vi "MainLoop.vi"() -> ()   [LabVIEW 2021]
uses:
  5a09477c-fa6a-4a2c-ae4e-0462b0b96a3d.vi
  6f825153-6f78-4197-a3b4-cb3bcc6ce098.vi
  <vilib>/DAQmx/read.llb/DAQmx Read (Digital 1D Bool 1Chan 1Samp).vi
  <vilib>/DAQmx/create/channels.llb/DAQmx Create Channel (DI-Digital Input).vi
  <vilib>/Utility/file.llb/Read Delimited Spreadsheet (DBL).vi
  GlobalSTATE.vi
  <vilib>/DAQmx/miscellaneous.llb/DAQmx Fill In Error Info.vi
  Global_BeamBreaks.vi
  <vilib>/Utility/file.llb/Write Delimited Spreadsheet (string).vi
panel:
  in  "stop":bool
  in  "Tab Control":enum32{"Settings", "Monitor", "Events"}(tab)
  in  "Task type":T1(ring)=enum."One drive changes"
  in  "Drive to change (in 'One drive changes')":enum32{"Food", "Water", "Social"}(ring)
  in  "Possible availability":i32[](array[numeric])=[0, 1, 2]
  in  "Control availability":i32=1
  in  "Beam break digital inputs":tag="Dev2/port0/line0:4"
  in  "Availability settings":i32[][](array[numeric])=[[0, 1, 2], [0, 1, 2], [0, 4000, 8000]]
  in  "file (use dialog)":path=path "C:/Code/Availability-maze-main/Availability-maze-main/MazeCode/LookUpTbl.txt"
  in  "Beam breaks":bool[](array[boolean])=[FALSE, FALSE, FALSE, FALSE, FALSE]
  out "Current State":string="CHOICE"
  out "Block length":i32=3
  out "Max pellets":u32
  out "Interaction time (ms)":u32=4000
  out "Max water drops":u32=1
  out "Block count":i32
  out "Trial of block":i32
  out "Food available":dbl(knob) scale=0.0..3.0
  out "Water available":dbl(knob)=0.46403176085318276 scale=0.0..3.0
  out "Social time available":dbl(knob)=4000.0 scale=0.0..10000.0
  out "serial comm":string="b"
  out "Event times":string[][](array[string])
  in  "Save event file?":bool
  in  "file path (dialog if empty)":path
  # "Low (0)     Medium (1)    High(2)"
  # "Pellets \n\nWater drops\n\nSocial time (ms)"
  # "Social                   Water                  Food               Middle             Home cage"
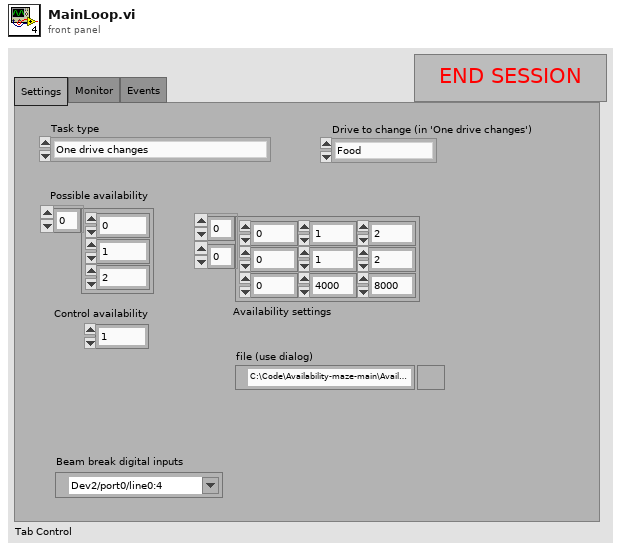
[diagram p1: front panel]
types:
  T1 = enum32{"All drives change and different", "One drive changes", "All drives same, but change"}
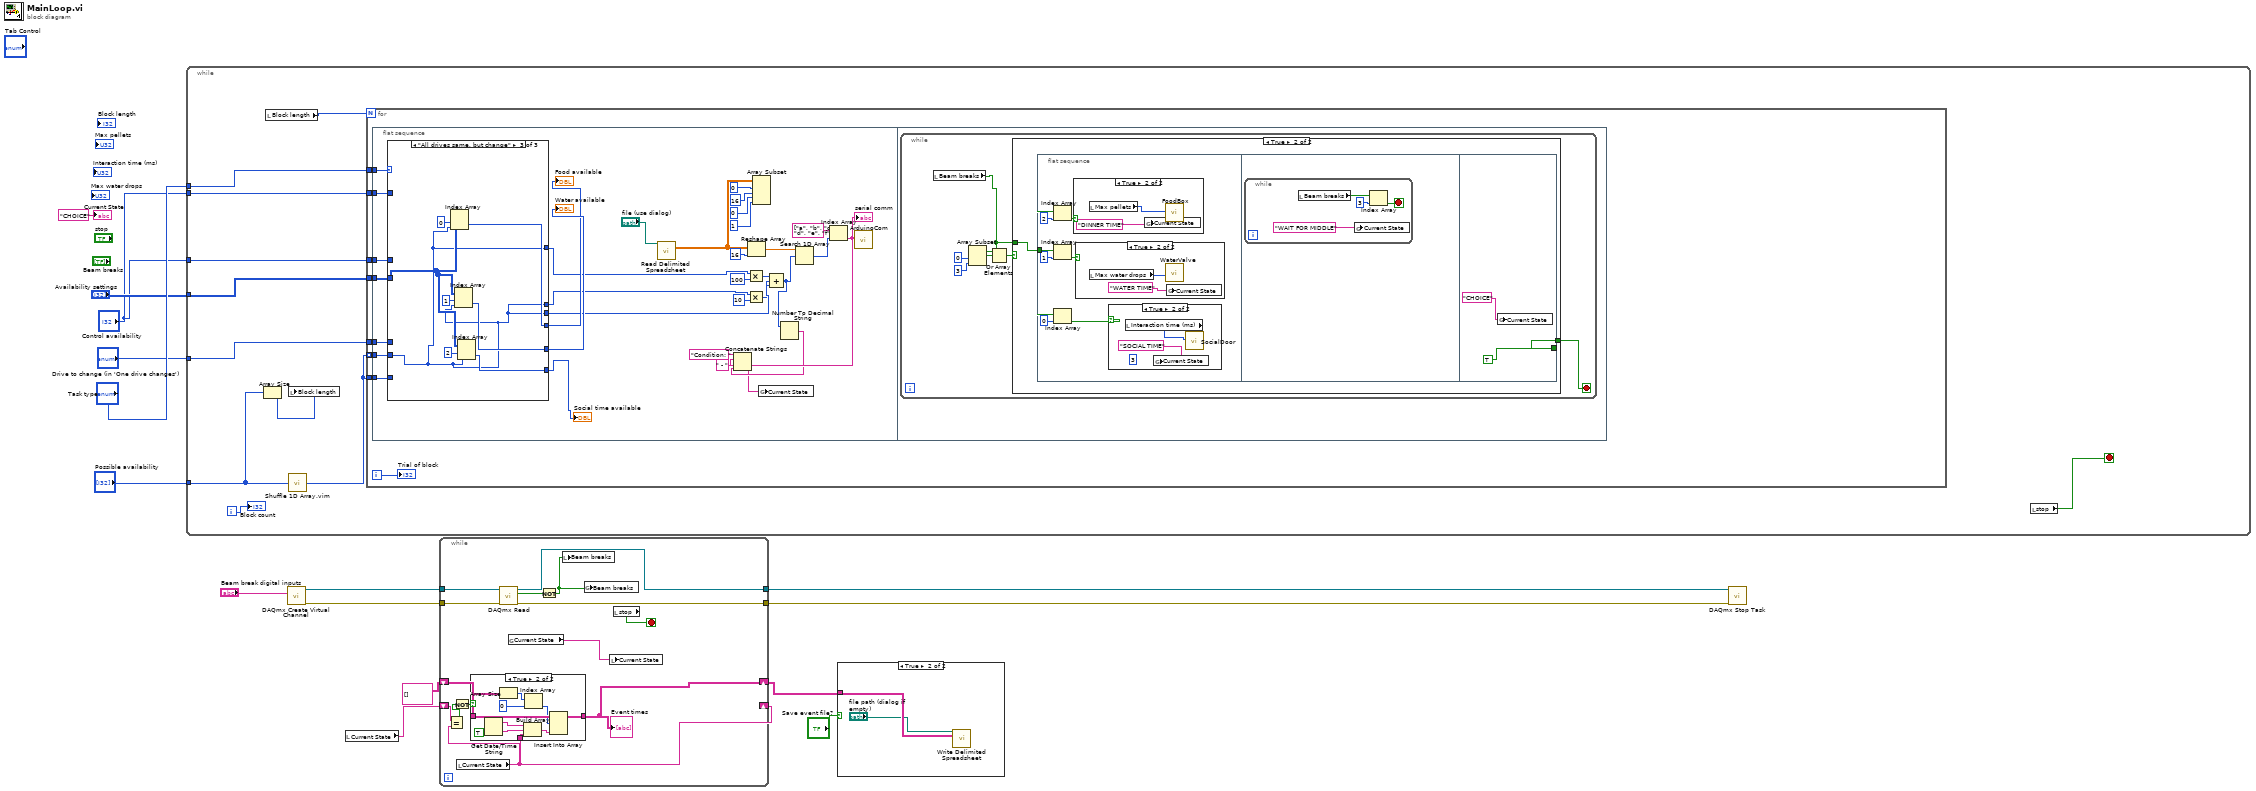
[diagram p0: block diagram]
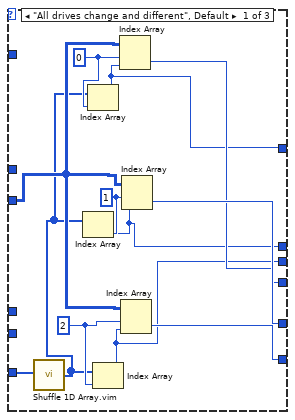
[diagram p4: hidden frame]
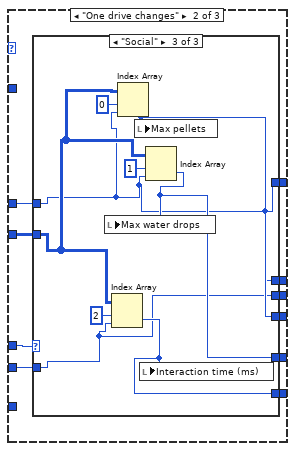
[diagram p5: hidden frame]
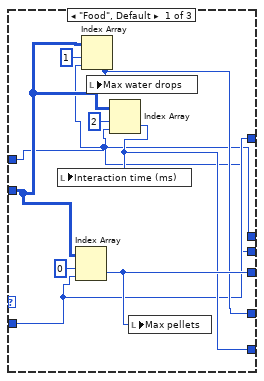
[diagram p6: hidden frame]
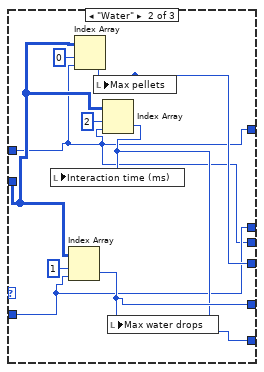
[diagram p7: hidden frame]
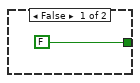
[diagram p8: hidden frame]
diagram:
  n1 = while {
    tunnel: "Task type" -> [w26]
    tunnel: "Drive to change (in 'One drive changes')" -> [w25]
    tunnel: "Possible availability" -> [w20]
    tunnel: "Availability settings" -> [w24]
    tunnel: "Control availability" -> [w23]
    tunnel: "Control availability" -> [w22]
    i -> [w18]
    stop <- w16 stop-if-true
    n2 = Array Size(array=w20) -> (size(s)=w19:i32)
    n3 = local read "Block length"() -> (w21:i32)
    n4 = local write "Block length"(w19) -> ()
    n5 = call "Shuffle 1D Array.vim"("array"=w20) -> ("shuffled array"=w17:i32[])  [unwired: 4 in]
    n6 = for {
      N: w21 -> [_]
      tunnel: w26 -> [w34]
      tunnel: w25 -> [w33]
      tunnel: w17 -> [w32] mode=indexing
      tunnel: w24 -> [w31]
      tunnel: w23 -> [w30]
      tunnel: w22 -> [w29]
      tunnel: w17 -> [w27]
      i -> [w28]
      n7 = flat-sequence {
        tunnel: w34 -> [w67]
        tunnel: w33 -> [w66]
        tunnel: w32 -> [w65]
        tunnel: w31 -> [w64]
        tunnel: w30 -> [w63]
        tunnel: w29 -> [w62]
        tunnel: w27 -> [w61]
        frame #0 {
          n8 = case shown="\"All drives same, but change\"" w67 {
            tunnel: w66 -> [_ w89 _]
            tunnel: w65 -> [_ w88 w117]
            tunnel: w64 -> [w79 w87 w121]
            tunnel: w63 -> [_ _ _]
            tunnel: w62 -> [_ w86 _]
            tunnel: [w71 w85 w120] -> w58
            tunnel: [w72 w84 w119] -> w60
            tunnel: [w76 w83 w118] -> w59
            tunnel: w61 -> [w78 _ _]
            tunnel: [w70 w82 w117] -> w55
            tunnel: [w69 w81 w117] -> w54
            tunnel: [w68 w80 w117] -> w53
            frame "All drives change and different", Default {
              w75 = 0 ("index")
              w74 = 1 ("index")
              w77 = 2 ("index")
              n9 = call "Shuffle 1D Array.vim"("array"=w78) -> ("shuffled array"=w73:i32[])  [unwired: 4 in]
              n10 = Index Array(array=w73, index=w74) -> (element=w69:i32)
              n11 = Index Array(array=w73, index=w75) -> (element=w70:i32)
              n12 = Index Array(array=w73, index=w77) -> (element=w68:i32)
              n13 = Index Array(array=w79, index (row)=w75, index (col)=w70) -> (element=w71:i32)
              n14 = Index Array(array=w79, index (row)=w77, index (col)=w68) -> (element=w76:i32)
              n15 = Index Array(array=w79, index (row)=w74, index (col)=w69) -> (element=w72:i32)
            }
            frame "One drive changes" {
              n16 = case shown="\"Social\"" w89 {
                tunnel: w88 -> [w91 w100 w108]
                tunnel: w87 -> [w95 w104 w113]
                tunnel: w86 -> [w90 w99 w109]
                tunnel: [w94 w103 w110] -> w85
                tunnel: [w93 w102 w112] -> w84
                tunnel: [w92 w101 w111] -> w83
                tunnel: [w91 w99 w109] -> w82
                tunnel: [w90 w100 w109] -> w81
                tunnel: [w90 w99 w108] -> w80
                frame "Food", Default {
                  n17 = Index Array(array=w95, index (row)=0 ("index"), index (col)=w91) -> (element=w94:i32)
                  n18 = Index Array(array=w95, index (row)=1, index (col)=w90) -> (element=w93:i32)
                  n19 = local write "Max water drops"(w93) -> ()
                  n20 = Index Array(array=w95, index (row)=2 ("disabled index (row)"), index (col)=w90) -> (element=w92:i32)
                  n21 = local write "Interaction time (ms)"(w92) -> ()
                  n22 = local write "Max pellets"(w94) -> ()
                }
                frame "Water" {
                  n23 = Index Array(array=w104, index (row)=1 ("index"), index (col)=w100) -> (element=w102:i32)
                  n24 = Index Array(array=w104, index (row)=0, index (col)=w99) -> (element=w103:i32)
                  n25 = local write "Max pellets"(w103) -> ()
                  n26 = Index Array(array=w104, index (row)=2 ("disabled index (row)"), index (col)=w99) -> (element=w101:i32)
                  n27 = local write "Interaction time (ms)"(w101) -> ()
                  n28 = local write "Max water drops"(w102) -> ()
                }
                frame "Social" {
                  n29 = Index Array(array=w113, index (row)=2 ("index"), index (col)=w108) -> (element=w111:i32)
                  n30 = Index Array(array=w113, index (row)=0, index (col)=w109) -> (element=w110:i32)
                  n31 = local write "Max pellets"(w110) -> ()
                  n32 = local write "Interaction time (ms)"(w111) -> ()
                  n33 = Index Array(array=w113, index (row)=1 ("disabled index (row)"), index (col)=w109) -> (element=w112:i32)
                  n34 = local write "Max water drops"(w112) -> ()
                }
              }
            }
            frame "All drives same, but change" {
              n35 = Index Array(array=w121, index (row)=0, index (col)=w117) -> (element=w120:i32)
              n36 = Index Array(array=w121, index (row)=1, index (col)=w117) -> (element=w119:i32)
              n37 = Index Array(array=w121, index (row)=2, index (col)=w117) -> (element=w118:i32)
            }
          }
          "Food available" <- w58
          "Water available" <- w60
          "Social time available" <- w59
          n38 = call-poly <vilib>:"Read Delimited Spreadsheet.vi"("file path (dialog if empty)"="file (use dialog)") -> ("all rows"=w44:dbl[][])  [unwired: 9 in, 5 out]
          n39 = Reshape Array(w44, 16 ("dimension size")) -> (w43:dbl[])
          n40 = Multiply(x=w55, y=100) -> (x*y=w51:i32)
          n41 = Multiply(x=w54, y=10) -> (x*y=w52:i32)
          n42 = Array Subset(array=w44, index (row)=0 ("index"), length (row)=16 ("length"), index (col)=0 ("index"), length (col)=1 ("length")) -> ()  [unwired: 1 out]
          n43 = Compound Arithmetic op=ADD(w51, w52, w53) -> (w37:i32)
          n44 = Number To Decimal String(number=w37) -> (decimal integer string=w36:string)  [unwired: 1 in]
          n45 = Search 1D Array(1D array=w43, element=w37) -> (index of element=w49:i32)  [unwired: 1 in]
          n46 = Index Array(array=string[] ["a", "b", "c", "d", "e", "f", "g", "h", "i", "j", "k", "l", "m", "n", "o"], index=w49) -> (element=w39:string)
          "serial comm" <- w39
          n47 = Concatenate Strings("Condition: " ("string"), w39, " - " ("string"), w36) -> (w35:string)
          n48 = global write "GlobalSTATE.vi" "Current State"(w35) -> ()
          n49 = call "ArduinoCom.vi"("write buffer"=w39) -> ()  [unwired: 11 in]
        }
        frame #1 {
          n50 = while {
            stop <- w125 stop-if-true
            n51 = local read "Beam breaks"() -> (w126:bool[])
            n52 = Array Subset(array=w126, index=0, length=3) -> (w129:bool[])
            n53 = Or Array Elements(Boolean array=w129) -> (logical OR=w130:bool)
            n54 = case shown="True" w130 {
              tunnel: w126 -> [_ w133]
              tunnel: [FALSE ("stop") w132] -> w125
              frame False {
              }
              frame True {
                n55 = flat-sequence {
                  tunnel: w133 -> [w134]
                  tunnel: [TRUE ("stop")] -> w132
                  frame #0 {
                    n56 = Index Array(array=w134, index=2) -> (element=w139:bool)
                    n57 = Index Array(array=w134, index=1) -> (element=w135:bool)
                    n58 = Index Array(array=w134, index=0) -> (element=w137:bool)
                    n59 = case shown="True" w139 {
                      frame False {
                      }
                      frame True {
                        n60 = local read "Max pellets"() -> (w146:u32)
                        n61 = global write "GlobalSTATE.vi" "Current State"("DINNER TIME" ("Current State")) -> ()
                        n62 = call "FoodBox.vi"("Max pellets"=w146) -> ()  [unwired: 10 in, 1 out]
                      }
                    }
                    n63 = case shown="True" w135 {
                      frame False {
                      }
                      frame True {
                        n64 = local read "Max water drops"() -> (w142:u32)
                        n65 = call "WaterValve.vi"("Max pulses"=w142) -> ()  [unwired: 11 in]
                        n66 = global write "GlobalSTATE.vi" "Current State"("WATER TIME" ("Current State")) -> ()
                      }
                    }
                    n67 = case shown="True" w137 {
                      frame False {
                      }
                      frame True {
                        (unwired) 3 ("index")
                        n68 = local read "Interaction time (ms)"() -> (w144:u32)
                        n69 = global write "GlobalSTATE.vi" "Current State"("SOCIAL TIME" ("Current State")) -> ()
                        n70 = call "SocialDoor.vi"("Interaction time"=w144) -> ()  [unwired: 11 in]
                      }
                    }
                  }
                  frame #1 {
                    n71 = while {
                      stop <- w148 stop-if-true
                      n72 = local read "Beam breaks"() -> (w149:bool[])
                      n73 = global write "GlobalSTATE.vi" "Current State"("WAIT FOR MIDDLE" ("Current State")) -> ()
                      n74 = Index Array(array=w149, index=3) -> (element=w148:bool)
                    }
                  }
                  frame #2 {
                    n75 = global write "GlobalSTATE.vi" "Current State"("CHOICE" ("Current State")) -> ()
                  }
                }
              }
            }
          }
        }
      }
      "Trial of block" <- w28
    }
    n76 = local read "stop"() -> (w16:bool)
    "Block count" <- w18
  }
  n77 = call-poly <vilib>:"DAQmx Create Virtual Channel.vi"("lines"="Beam break digital inputs") -> ("task out"=w14:refnum<k21>, "error out"=w13:errorcluster)  [unwired: 13 in]
  n78 = local read "Current State"() -> (w3:string)
  n79 = while {
    tunnel: w14 -> [w165]
    tunnel: w13 -> [w164]
    tunnel: [w163] -> w12
    tunnel: [w162] -> w11
    shift-right: [w156] -> w2
    shift-left: string[][] [] -> [w157]
    shift-right: [w155] -> _
    shift-left: w3 -> [w154]
    stop <- w161 stop-if-true
    n80 = local read "Current State"() -> (w155:string)
    n81 = Equal?(x=w154, y=w155) -> (x = y?=w158:bool)
    n82 = Not(x=w158) -> (.not. x?=w159:bool)
    n83 = case shown="True" w159 {
      tunnel: w157 -> [w167 w177]
      tunnel: [w167 w176] -> w156
      tunnel: w155 -> [_ w171]
      frame False {
      }
      frame True {
        n84 = Get Date/Time String(want seconds? (F)=TRUE) -> (date string=w169:string, time string=w170:string)  [unwired: 2 in]
        n85 = Array Size(array=w177) -> (size(s)=w175:i32[])
        n86 = Build Array(w169, w170, w171) -> (w172:string[])
        n87 = Index Array(array=w175, index=0) -> (element=w173:i32)
        n88 = Insert Into Array(array=w177, index (row)=w173, new element=w172) -> (w176:string[][])  [unwired: 1 in]
      }
    }
    "Event times" <- w156
    n89 = call-poly <vilib>:"DAQmx Read.vi"("task/channels in"=w165, "error in"=w164) -> ("task out"=w163:refnum<k21>, "data"=w166:bool[], "error out"=w162:errorcluster)  [unwired: 11 in]
    n90 = global read "GlobalSTATE.vi" "Current State"() -> (w153:string)
    n91 = Not(x=w166) -> (.not. x?=w160:bool[])
    n92 = local write "Beam breaks"(w160) -> ()
    n93 = global write "Global_BeamBreaks.vi" "Beam breaks"(w160) -> ()
    n94 = local write "Current State"(w153) -> ()
    n95 = local read "stop"() -> (w161:bool)
  }
  n96 = case shown="True" "Save event file?" {
    tunnel: w2 -> [_ w179]
    frame False {
    }
    frame True {
      n97 = call-poly <vilib>:"Write Delimited Spreadsheet.vi"("file path (dialog if empty)"="file path (dialog if empty)", "2D data"=w179) -> ()  [unwired: 12 in, 2 out]
    }
  }
  n98 = call <vilib>:"DAQmx Stop Task.vi"("task/channels in"=w12, "error in"=w11) -> ()  [unwired: 12 in, 2 out]
  "Current State" <- "CHOICE" ("Current State")
